vi "Change_Temp.vi"() -> ()   [LabVIEW 2015]
panel:
  out "error out":errorcluster
  in  "Temp":string
  in  "IP":string
  in  "Port":string
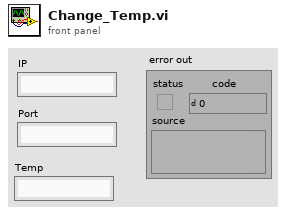
[diagram p1: front panel]
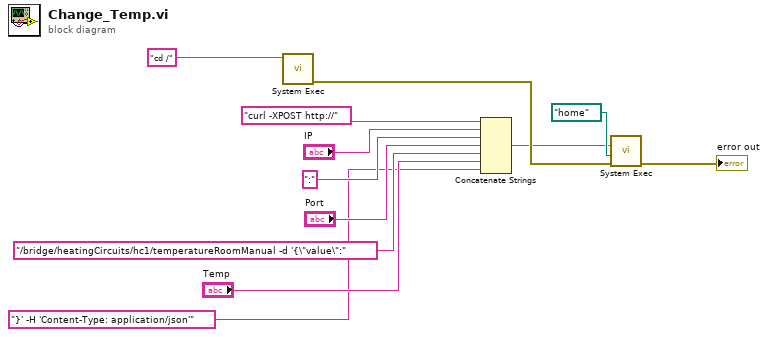
[diagram p0: block diagram]
diagram:
  n1 = call <vilib>:"System Exec.vi"("command line"="cd /") -> ("error out"=w11:errorcluster)  [unwired: 7 in, 3 out]
  n2 = Concatenate Strings("curl -XPOST http://" ("string"), "IP", ":" ("string"), "Port", "/bridge/heatingCircuits/hc1/temperatureRoomManual -d '{\"value\":" ("string"), "Temp", "}' -H 'Content-Type: application/json'" ("string")) -> (w1:string)
  n3 = call <vilib>:"System Exec.vi"("error in (no error)"=w11, "working directory"=path "/home", "command line"=w1) -> ("error out"=→"error out":errorcluster)  [unwired: 5 in, 3 out]
